vi "test_Add Local Chassis.vi"(8 "error in (no error)":errorcluster, 11 "TestCase in":refnum<class "Scan Engine Scripting API Custom Device Unit Tests.lvclass">) -> (0 "error out":errorcluster, 3 "TestCase out":refnum<class "Scan Engine Scripting API Custom Device Unit Tests.lvclass">)   [LabVIEW 2020, in "Scan Engine Scripting API Custom Device Unit Tests.lvclass"]
uses:
  Scan Engine Scripting API Custom Device Unit Tests.lvclass
  Scan Engine Scripting API Custom Device Unit Tests.lvclass/Scan Engine Scripting API Custom Device Unit Tests.ctl
  <vilib>/Addons/_JKI Toolkits/VI Tester/TestCase.llb/TestCase.lvclass
  Scripting/Scan Engine Scripting.lvlib
  Shared/Type Defs/Main Settings.ctl
  Shared/SEECD Shared.lvlib
  Shared/Type Defs/Local Chassis Settings.ctl
  C:/Users/Administrator/Desktop/Jatin/All DNC DLLs/NationalInstruments.VeriStand.SystemDefinitionAPI.dll
  Jatin/All DNC DLLs/NationalInstruments.VeriStand.SystemDefinitionAPI.dll
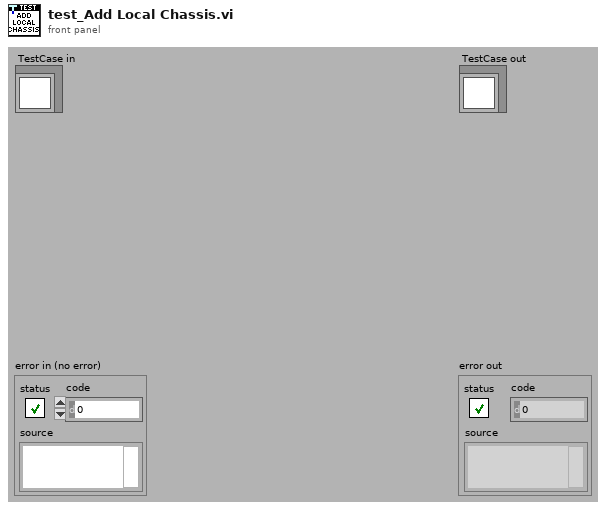
[diagram p1: front panel]
types:
  T1 = typedef "SEECD Shared.lvlib/Local Chassis Settings.ctl" = cluster{"name":string, "number of slots":i32}
  T2 = typedef "SEECD Shared.lvlib/Main Settings.ctl" = cluster{"sync to scan":bool, "scan engine decimation":u16, "delay after FPGA load (s)":u16}
  T3 = typedef "Custom Device API.lvlib/Custom Device Item Ref.ctl" = u64
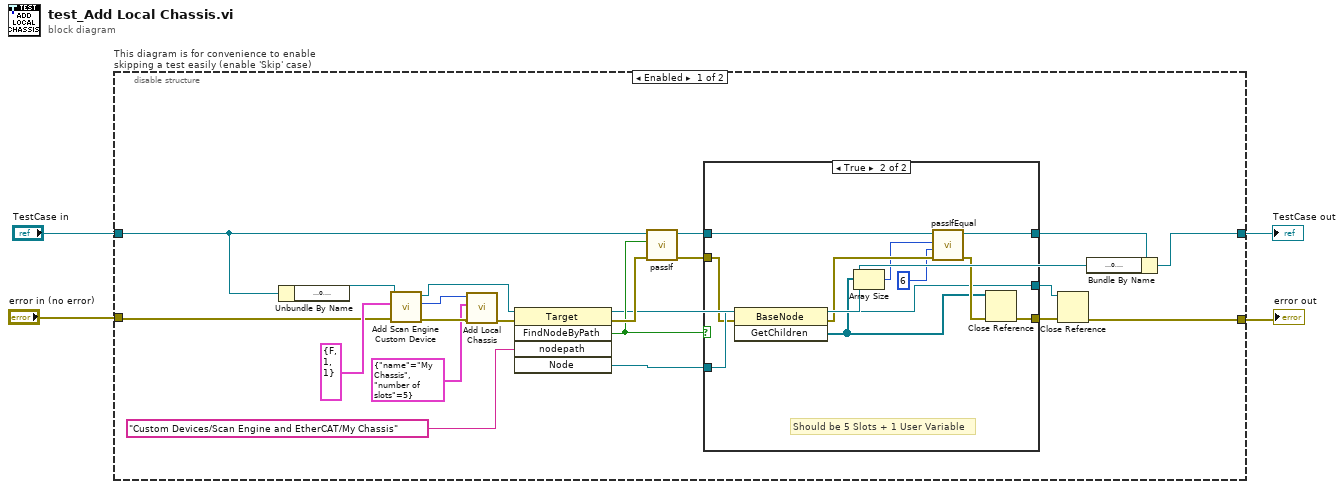
[diagram p0: block diagram]
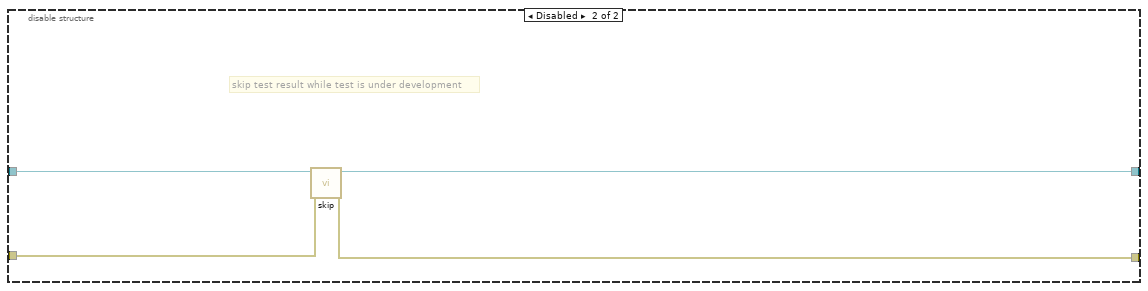
[diagram p3: hidden frame]
diagram:
  n1 = disable-structure "This diagram is for convenience to enable skipping a test easily (enable 'Skip' case)" shown="Enabled" {
    disable-tunnel: "TestCase in" -> [w11 w43]
    disable-tunnel: [w5 w41] -> w1
    disable-tunnel: [w6 w42] -> w3
    disable-tunnel: "error in (no error)" -> [w10 w40]
    frame Enabled {
      n2 = Unbundle By Name(w11) -> ("target ref"=w9:refnum<k24>)
      n3 = call "Add Scan Engine Custom Device.vi"("error in"=w10, "settings"=T2 {"sync to scan"=FALSE, "scan engine decimation"=1, "delay after FPGA load (s)"=1}, "NationalInstruments.VeriStand.SystemDefinitionAPI.Target"=w9) -> ("error out"=w24:errorcluster, "scan engine custom device ref"=w23:T3, "NationalInstruments.VeriStand.SystemDefinitionAPI.Target"=w21:refnum<k39>)  [unwired: 6 in]
      n4 = call "Add Local Chassis.vi"("error in"=w24, "settings"=T1 {"name"="My Chassis", "number of slots"=5}, "scan engine custom device ref in"=w23) -> ("error out"=w13:errorcluster)  [unwired: 4 in, 4 out]
      n5 = invoke class="Target" method="FindNodeByPath"(reference=w21, error in=w13, "nodepath"="Custom Devices/Scan Engine and EtherCAT/My Chassis") -> (reference out=w7:refnum<k39>, error out=w20:errorcluster, "FindNodeByPath"=w19:bool, "Node"=w16:refnum<k39>)  [unwired: 2 in, 1 out]
      n6 = call-dynamic "passIf.vi"("error in (no error)"=w20, "pass"=w19, "TestCase in"=w11) -> ("error out"=w18:errorcluster, "TestCase out"=w17:refnum<class "Scan Engine Scripting API Custom Device Unit Tests.lvclass">)  [unwired: 7 in]
      n7 = case shown="True" w19 {
        tunnel: w18 -> [w27 w38]
        tunnel: w17 -> [w28 w37]
        tunnel: w16 -> [w26 w39]
        tunnel: [w28 w33] -> w8
        tunnel: [w27 w30] -> w15
        tunnel: [w26 w29] -> w14
        frame False {
        }
        frame True {
          # "Should be 5 Slots + 1 User Variable"
          n8 = invoke class="BaseNode" method="GetChildren"(reference=w39, error in=w38) -> (reference out=w29:refnum<k39>, error out=w36:errorcluster, "GetChildren"=w31:refnum<k39>[])  [unwired: 1 in]
          n9 = Array Size(array=w31) -> (size(s)=w35:i32)
          n10 = call-dynamic "passIfEqual.vi"("error in (no error)"=w36, "y"=6 ("size(s)"), "x"=w35, "TestCase in"=w37) -> ("error out"=w32:errorcluster, "TestCase out"=w33:refnum<class "Scan Engine Scripting API Custom Device Unit Tests.lvclass">)  [unwired: 6 in]
          n11 = Close Reference(reference=w31, error in (no error)=w32) -> (error out=w30:errorcluster)
        }
      }
      n12 = Close Reference(reference=w14, error in (no error)=w15) -> (error out=w6:errorcluster)
      n13 = Bundle By Name(cluster=w8, "target ref"=w7) -> (w5:refnum<class "Scan Engine Scripting API Custom Device Unit Tests.lvclass">)
    }
    frame Disabled {
      # "skip test result while test is under development"
      n14 = call <vilib>:"skip.vi"("error in (no error)"=w40, "TestCase in"=w43) -> ("error out"=w42:errorcluster, "TestCase out"=w41:refnum<class "Scan Engine Scripting API Custom Device Unit Tests.lvclass">)  [unwired: 8 in]
    }
  }
  "error out" <- w3
  "TestCase out" <- w1
